vi "execute.vi"(10 "task token":refnum<class "null task token.lvclass">, 11 "action in":refnum<class "action.lvclass">) -> (3 "result":refnum<class "result.lvclass">)   [LabVIEW 2013, in "action.lvclass"]
uses:
  action.lvclass
  result/result.lvclass
  task token/null task token.lvclass
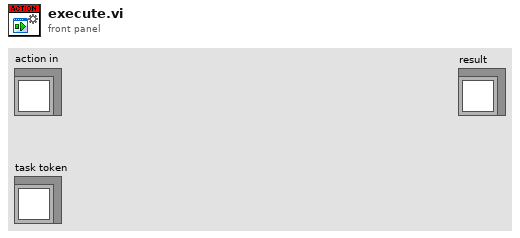
[diagram p1: front panel]
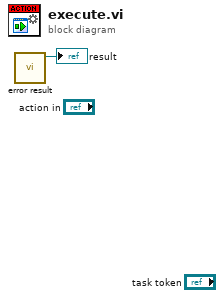
[diagram p0: block diagram]
diagram:
  n1 = call "error result.vi"() -> ("result"=→"result":refnum<class "result.lvclass">)  [unwired: 11 in]
